vi "AWS-S3-GenerateExpiringLink.vi"(0 "AWS-S3-API":refnum<class "AWS-S3-API.lvclass">, 1 "Verb":i32(ring) items=["GET", "HEAD", "PUT", "DELETE"], 5 "Object Bucket":string, 7 "Object Key":string, 9 "Expires":timestamp, 11 "error in":errorcluster) -> (4 "AWS-S3-API out":refnum<class "AWS-S3-API.lvclass">, 6 "Pre-Signed URL":string, 15 "error out":errorcluster)   [LabVIEW 2012, in "AWS-S3-API.lvclass"]
uses:
  AWS-S3-API.lvclass
  C:/Users/Jack/repo/visualize/Dependencies/aws/AWS-SDK/AWSSDK.dll
  AWS-SDK/AWSSDK.dll
panel:
  # "Inputs"
  # "Outputs"
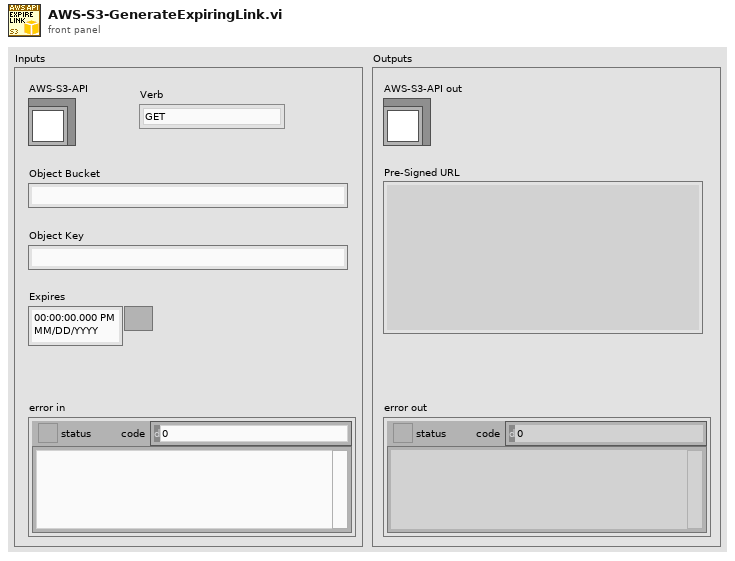
[diagram p1: front panel]
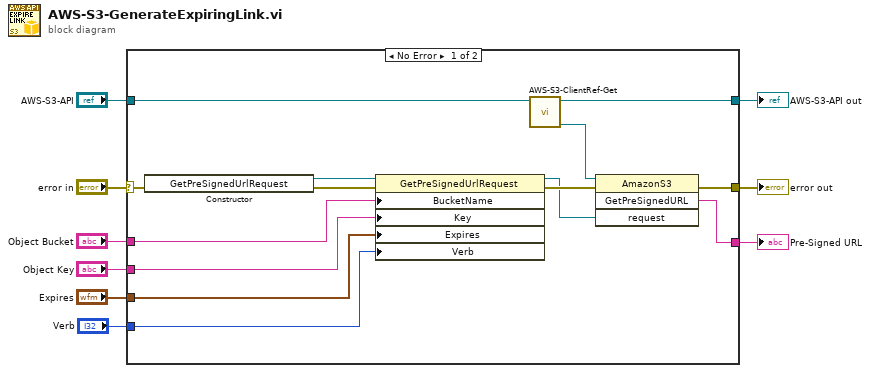
[diagram p0: block diagram]
diagram:
  n1 = case shown="No Error" "error in" {
    selector: "error in" -> [w20 w25]
    tunnel: [w23 w25] -> w9
    tunnel: [w10 w24] -> w7
    tunnel: "AWS-S3-API" -> [w11 w24]
    tunnel: [w22 _] -> w5
    tunnel: "Expires" -> [w18 _]
    tunnel: "Object Key" -> [w17 _]
    tunnel: "Object Bucket" -> [w16 _]
    tunnel: "Verb" -> [w15 _]
    frame No Error {
      n2 = constructor class="GetPreSignedUrlRequest"(error in=w20) -> (reference out=w21:refnum<k24>, error out=w19:errorcluster)  [unwired: 2 in, 1 out]
      n3 = property class="GetPreSignedUrlRequest"(reference=w21, error in=w19, "BucketName"=w16, "Key"=w17, "Expires"=w18, "Verb"=w15) -> (reference out=w13:refnum<k24>, error out=w14:errorcluster)
      n4 = call "AWS-S3-ClientRef-Get.vi"("AWS-S3-API"=w11) -> ("S3 Client ref"=w12:refnum<k24>, "AWS-S3-API out"=w10:refnum<class "AWS-S3-API.lvclass">)  [unwired: 9 in]
      n5 = invoke class="AmazonS3" method="GetPreSignedURL"(reference=w12, error in=w14, "request"=w13) -> (error out=w23:errorcluster, "GetPreSignedURL"=w22:string)  [unwired: 1 in, 2 out]
    }
    frame Error {
    }
  }
  "error out" <- w9
  "AWS-S3-API out" <- w7
  "Pre-Signed URL" <- w5
